vi "设置模块队列名.vi"() -> (2 "Msg":string)   [LabVIEW 2022 SP3, in "斯坦道氨氮V2.lvlib"]
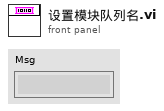
[diagram p1: front panel]
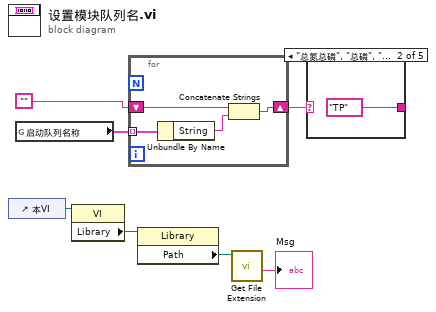
[diagram p0: block diagram]
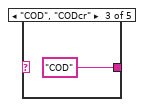
[diagram p3: hidden frame]
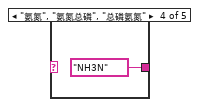
[diagram p4: hidden frame]
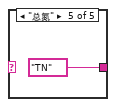
[diagram p5: hidden frame]
diagram:
  n1 = control-ref of="本VI"() -> (w3:refnum<vi>)
  n2 = global read "总磷总氮断电保存全局变量.vi" "启动队列名称"() -> (w6:cluster{"String":string, "Value":u16}[])
  n3 = property class="VI"(reference=w3) -> ("Library"=w4:refnum<vi>)  [unwired: 1 in, 2 out]
  n4 = for {
    tunnel: w6 -> [w11] mode=indexing
    shift-right: [w10] -> w5
    shift-left: "" -> [w8]
    n5 = Unbundle By Name(w11) -> ("String"=w9:string)
    n6 = Concatenate Strings(w8, w9) -> (w10:string)
  }
  n7 = property class="Library"(reference=w4) -> ("Path"=w2:path)  [unwired: 1 in, 2 out]
  n8 = call <vilib>:"Get File Extension.vi"("file"=w2) -> ("filename without extension"=→"Msg":string)  [unwired: 6 in, 4 out]
  n9 = case shown="\"总氮总磷\", \"总磷\", \"总磷总氮\"" w5 {
    selector: w5 -> [w12 _ _ _ _]
    tunnel: [w12 "TP" ("队列名") "COD" ("队列名") "NH3N" ("队列名") "TN" ("队列名")] -> _
    frame Default {
    }
    frame "总氮总磷", "总磷", "总磷总氮" {
    }
    frame "COD", "CODcr" {
    }
    frame "氨氮", "氨氮总磷", "总磷氨氮" {
    }
    frame "总氮" {
    }
  }
